vi "Demo Input server.vi"(8 "error in (no error)":errorcluster) -> (0 "error out":errorcluster, 3 "Numeric":i32)   [LabVIEW 2013]
doc: "reentrant"
uses:
  VIremote.llb/VIremoteEvent.ctl
  VIremote.llb/VIremoteFunction.ctl
panel:
  in  "VIremoteEvent":T1
  out "change":bool
  in  "-":bool
  in  "+":bool
  in  "Combo Box iPad Test":string(combo)="First Combo Box element"
  in  "next":bool
  in  "String":string="Tap here"
  # "The up/down buttons will not work without mouse emulation but you can always make your own. Tap the numeric inicator to diplay popup to change its value via keyboard or slider (on iOS 5 also up-down buttons). All changes will be signaled."
  # "Connect two devices at the same time and see that they have their own data."
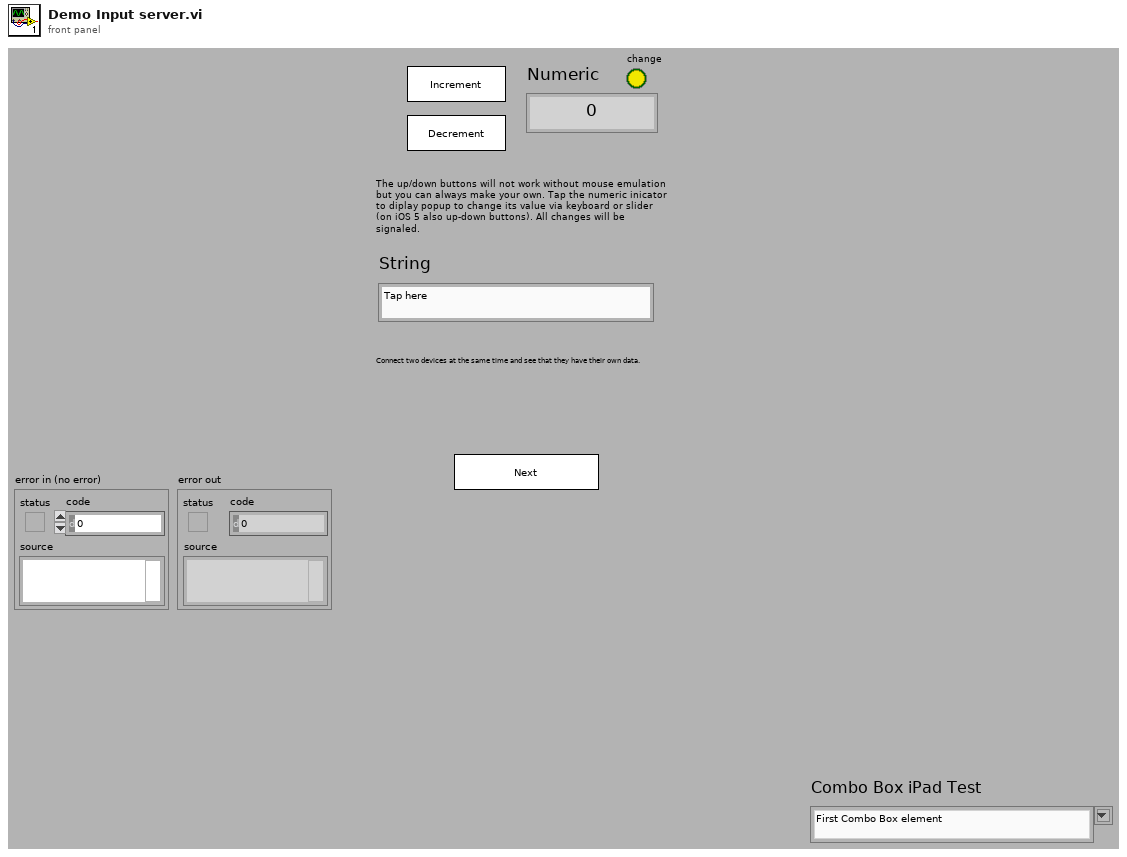
[diagram p1: front panel]
types:
  T1 = typedef "VIremoteEvent.ctl" = enum16{"No Event", "Connection Closed", "Navigate Back", "Enter Background", "Enter Foreground", "Portrait", "Portrait Upside Down", "Landscape Left", "Landscape Right"}
  T2 = typedef "VIremoteFunction.ctl" = enum16{"Do nothing", "Stop controller", "Close this connection", "Show info panel", "Set VI to control", "Set Accelerometer freq (Hz)", "Show Alert message", "Start Sound Input", "Stop Sound Input", "Set Volume (0-100)", "Set sound output Speaker", "Set sound output Receiver", "Play Sound", "Repeat Sound", "Stop Sound", "Pause Sound", "Resume Sound", "Set panel width of caller (320 or 480)", "Set Panel Size to Portrait", "Set Panel Size to Landscape", "Set Panel Size as Current Orientation", "Allow all UI Orientations", "Send user notification", "Disable Scrolling", "Normal Scrolling", "Page Scrolling", "Set Scroll Offset", "Page Indicator Position"}
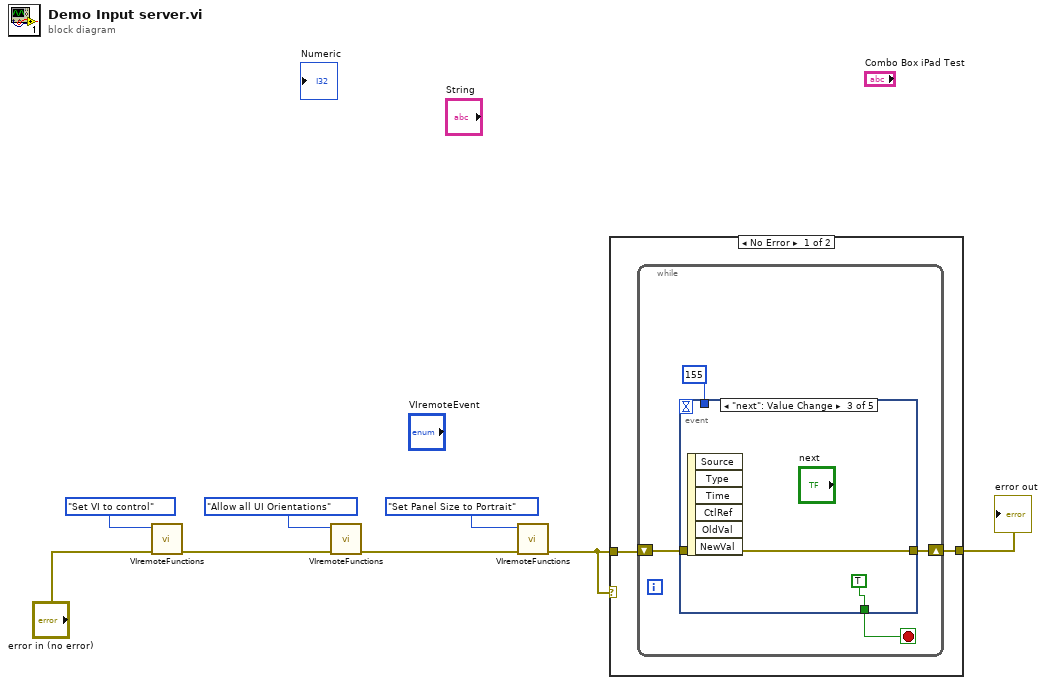
[diagram p0: block diagram]
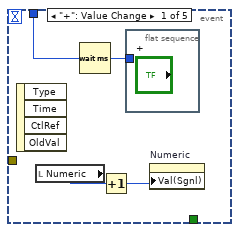
[diagram p2: hidden frame]
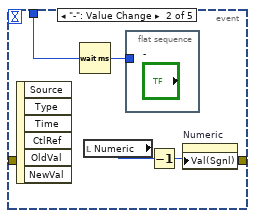
[diagram p3: hidden frame]
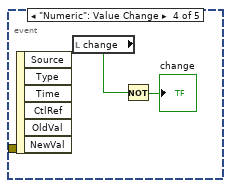
[diagram p4: hidden frame]
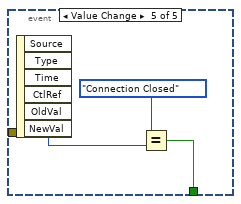
[diagram p5: hidden frame]
diagram:
  n1 = call "VIremoteFunctions.vi"("error in (no error)"="error in (no error)", "Function"=VIremoteFunction."Set VI to control") -> ("error out"=w4:errorcluster)  [unwired: 4 in, 5 out]
  n2 = call "VIremoteFunctions.vi"("error in (no error)"=w4, "Function"=VIremoteFunction."Allow all UI Orientations") -> ("error out"=w6:errorcluster)  [unwired: 4 in, 5 out]
  n3 = call "VIremoteFunctions.vi"("error in (no error)"=w6, "Function"=VIremoteFunction."Set Panel Size to Portrait") -> ("error out"=w1:errorcluster)  [unwired: 4 in, 5 out]
  n4 = case shown="No Error" w1 {
    tunnel: w1 -> [w10 w30]
    tunnel: [w9 w30] -> w2
    frame No Error {
      n5 = while {
        shift-right: [w12] -> w9
        shift-left: w10 -> [w13]
        stop <- w14 stop-if-true
        n6 = event shown="[2] \"next\": Value Change" {
          selector: _ -> [_ _ _ _ _]
          dyn-events: _ -> [_ _ _ _ _]
          timeout: _ -> [_ _ _ _ _]
          tunnel: [_ _ TRUE _ w27] -> w14
          tunnel: w13 -> [_ _ w23 _ _]
          tunnel: [_ _ w23 _ _] -> w12
          tunnel: u32 155 ("milliseconds to wait") -> [w17 w21 _ _ _]
          event "+": Value Change {
            n7 = event-data() -> ()  [unwired: 5 out]
            n8 = local read "Numeric"() -> (w18:i32)
            n9 = Wait (ms)(milliseconds to wait=w17) -> (millisecond timer value=w16:u32)
            n10 = Increment(x=w18) -> (x+1=w15:i32)
            n11 = flat-sequence {
              tunnel: w16 -> [_]
              frame #0 {
              }
            }
            n12 = property on="Numeric" class="DigNum (strict)"("Val(Sgnl)"=w15) -> ()  [unwired: 2 in, 2 out]
          }
          event "-": Value Change {
            n13 = event-data() -> ()  [unwired: 7 out]
            n14 = Wait (ms)(milliseconds to wait=w21) -> (millisecond timer value=w20:u32)
            n15 = local read "Numeric"() -> (w22:i32)
            n16 = flat-sequence {
              tunnel: w20 -> [_]
              frame #0 {
              }
            }
            n17 = Decrement(x=w22) -> (x-1=w19:i32)
            n18 = property on="Numeric" class="DigNum (strict)"("Val(Sgnl)"=w19) -> ()  [unwired: 2 in, 2 out]
          }
          event "next": Value Change {
            n19 = event-data() -> ()  [unwired: 7 out]
          }
          event "Numeric": Value Change {
            n20 = event-data() -> ()  [unwired: 7 out]
            n21 = local read "change"() -> (w25:bool)
            n22 = Not(x=w25) -> (.not. x?=→"change":bool)
          }
          event Value Change {
            n23 = event-data() -> ("NewVal"=w28:T1)  [unwired: 6 out]
            n24 = Equal?(x=VIremoteEvent."Connection Closed" ("VIremoteEvent"), y=w28) -> (x = y?=w27:bool)
          }
        }
      }
    }
    frame Error {
    }
  }
  "error out" <- w2
